vi "libremove_output.vi"(8 "error in (no error)":errorcluster, 11 "output":i32) -> (0 "error out":errorcluster)   [LabVIEW 2015]
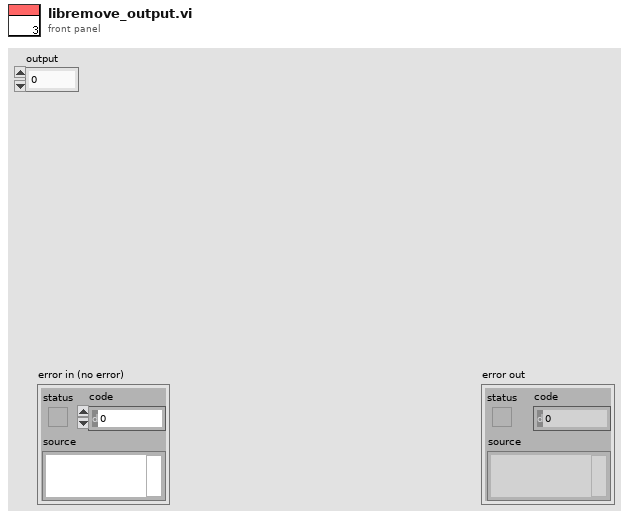
[diagram p1: front panel]
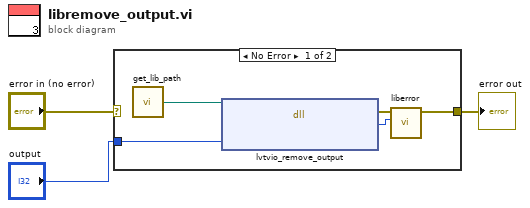
[diagram p0: block diagram]
diagram:
  n1 = case shown="No Error" "error in (no error)" {
    selector: "error in (no error)" -> [_ w9]
    tunnel: [w4 w9] -> w2
    tunnel: "output" -> [w7 _]
    frame No Error {
      n2 = call "get_lib_path.vi"() -> ("Path"=w8:path)
      n3 = dll-call lib="S:/thingiverselv/lib/liblvtvio.dll" fn="lvtvio_remove_output"(path in=w8, "output"=w7) -> (error out=w5:errorcluster, "return type"=w6:i32)  [unwired: 3 in, 1 out]
      n4 = call "liberror.vi"("tvio errors"=w6, "error in (no error)"=w5) -> ("error out"=w4:errorcluster)  [unwired: 9 in]
    }
    frame Error {
    }
  }
  "error out" <- w2
